vi "Is Empty.vi"(4 "JSON":string) -> (1 "Empty":bool)   [LabVIEW 2019, in "JSONtext.lvlib"]
doc: "Returns TRUE if the input text starts with any of these JSON types that are \"empty\":\n1) null\n2) NaN\n3) \"\" (an empty JSON string)\n4) A JSON Object containing no items\n5) An empty JSON Array \n6) no JSON at all (empty string or only whitespace)\n\nReturns False if the input starts with non-empty JSON.\n\nThis function will return FALSE if it detects invalid JSON, but as it only inspects the lead characters, it cannot be relied on to validate the input as proper JSON."
uses:
  JSONtext.lvlib
  Parsing/Advance past Line Ending.vi
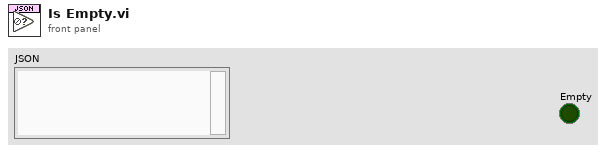
[diagram p1: front panel]
types:
  T1 = typedef "JSONtext.lvlib/JSON Value Type.ctl" = enum16{"Not a JSON Value", "JSON Object", "JSON Array", "String", "Number", "true", "false", "null"}
  T2 = typedef "JSONtext.lvlib/Parsing State.ctl" = enum16{"Parser Error", "Object", "Array", "String", "Number/Other", "Leading Whitespace", "Object end", "Array end", "Value end"}
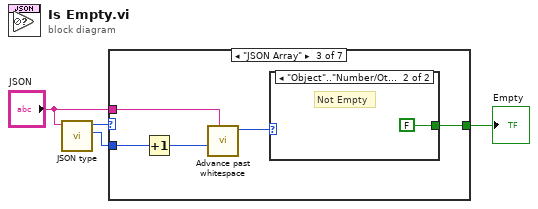
[diagram p0: block diagram]
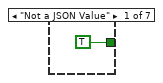
[diagram p2: hidden frame]
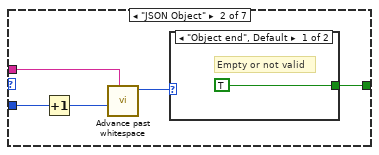
[diagram p3: hidden frame]
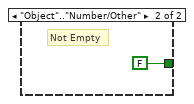
[diagram p4: hidden frame]
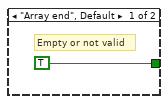
[diagram p5: hidden frame]
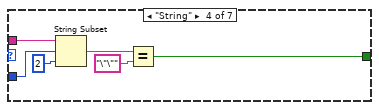
[diagram p6: hidden frame]
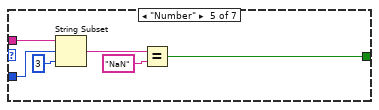
[diagram p7: hidden frame]
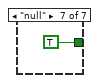
[diagram p9: hidden frame]
diagram:
  n1 = call "JSON type.vi"("JSON"="JSON") -> ("Item Offset"=w3:i32, "JSON Value Type"=w4:T1)  [unwired: 9 in]
  n2 = case shown="\"JSON Array\"" w4 {
    tunnel: w3 -> [_ w10 w17 w24 w30 _ _]
    tunnel: "JSON" -> [_ w9 w16 w25 w31 _ _]
    tunnel: [TRUE w6 w13 w21 w27 _ TRUE] -> w1
    frame "Not a JSON Value" {
    }
    frame "JSON Object" {
      n3 = Increment(x=w10) -> (x+1=w8:i32)
      n4 = call "Advance past whitespace.vi"("JSON"=w9, "Offset"=w8) -> ("Parser State"=w7:T2)  [unwired: 7 in, 2 out]
      n5 = case shown="\"Object end\", Default" w7 {
        tunnel: [TRUE FALSE] -> w6
        frame "Object end", Default {
          # "Empty or not valid"
        }
        frame "Object".."Number/Other" {
          # "Not Empty"
        }
      }
    }
    frame "JSON Array" {
      n6 = Increment(x=w17) -> (x+1=w15:i32)
      n7 = call "Advance past whitespace.vi"("JSON"=w16, "Offset"=w15) -> ("Parser State"=w14:T2)  [unwired: 7 in, 2 out]
      n8 = case shown="\"Object\"..\"Number/Other\"" w14 {
        tunnel: [TRUE FALSE] -> w13
        frame "Array end", Default {
          # "Empty or not valid"
        }
        frame "Object".."Number/Other" {
          # "Not Empty"
        }
      }
    }
    frame "String" {
      n9 = String Subset(string=w25, offset (0)=w24, length (rest)=2 ("length (rest)")) -> (substring=w23:string)
      n10 = Equal?(x=w23, y="\"\"") -> (x = y?=w21:bool)
    }
    frame "Number" {
      n11 = String Subset(string=w31, offset (0)=w30, length (rest)=3 ("length (rest)")) -> (substring=w29:string)
      n12 = Equal?(x=w29, y="NaN") -> (x = y?=w27:bool)
    }
    frame "true", "false" {
    }
    frame "null" {
    }
  }
  "Empty" <- w1
